vi "Eat Whitespace.vi"(8 "error in (no error)":errorcluster, 10 "Index In":i32, 11 "JSON String":string) -> (0 "error out":errorcluster, 2 "Index Out":i32, 3 "JSON String Passthrough":string)   [LabVIEW 2017, in "Advanced Variant Tools.lvlib" / "JSON.lvlib"]
uses:
  JSON/JSON.lvlib
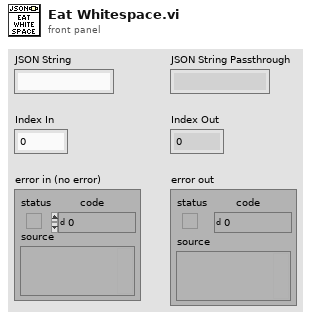
[diagram p1: front panel]
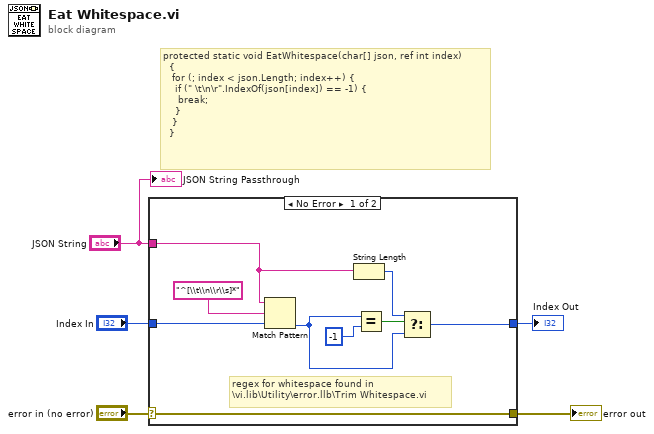
[diagram p0: block diagram]
diagram:
  # "protected static void EatWhitespace(char[] json, ref int index)\n\t\t{\n\t\t\tfor (; index < json.Length; index++) {\n\t\t\t\tif (\" \\t\\n\\r\".IndexOf(json[index]) == -1) {\n\t\t\t\t\tbreak;\n\t\t\t\t}\n\t\t\t}\n\t\t}"
  n1 = case shown="No Error" "error in (no error)" {
    selector: "error in (no error)" -> [w10 w16]
    tunnel: [w10 w16] -> w4
    tunnel: "JSON String" -> [w8 _]
    tunnel: "Index In" -> [w7 w15]
    tunnel: [w6 w15] -> w2
    frame No Error {
      # "regex for whitespace found in \n\\vi.lib\\Utility\\error.llb\\Trim Whitespace.vi"
      n2 = Match Pattern(string=w8, regular expression="^[\\t\\n\\r\\s]*", offset (0)=w7) -> (offset past match=w9:i32)  [unwired: 3 out]
      n3 = String Length(string=w8) -> (length=w11:i32)
      n4 = Equal?(x=w9, y=-1) -> (x = y?=w13:bool)
      n5 = Select(t=w11, s=w13, f=w9) -> (s? t:f=w6:i32)
    }
    frame Error {
    }
  }
  "error out" <- w4
  "Index Out" <- w2
  "JSON String Passthrough" <- "JSON String"
